vi "user event out globals - SubVI.vi"() -> ()   [LabVIEW 2014]
uses:
  Move stage command - Global - SubVI.ctl
panel:
  out "user event out":refnum<user-event>
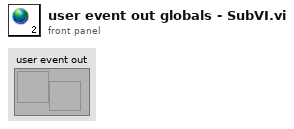
[diagram p1: front panel]
diagram:
